vi "Temperature Feedback.vi"(10 "Temp Array":dbl[](array[numeric]), 11 "input cluster":T1) -> (3 "Change in Reactivity":dbl)   [LabVIEW 2019]
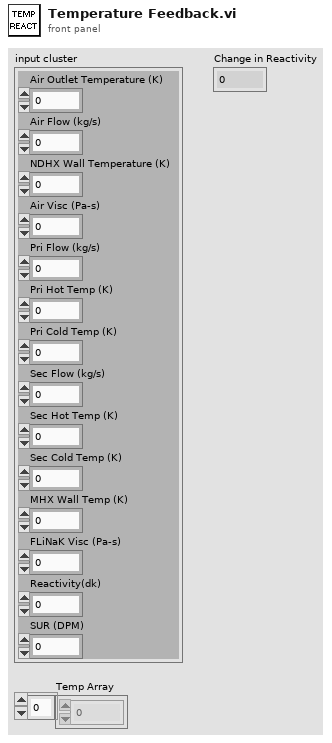
[diagram p1: front panel]
types:
  T1 = cluster{"Air Outlet Temperature (K)":dbl, "Air Flow (kg/s)":dbl, "NDHX Wall Temperature (K)":dbl, "Air Visc (Pa-s)":dbl, "Pri Flow (kg/s)":dbl, "Pri Hot Temp (K)":dbl, "Pri Cold Temp (K)":dbl, "Sec Flow (kg/s)":dbl, "Sec Hot Temp (K)":dbl, "Sec Cold Temp (K)":dbl, "MHX Wall Temp (K)":dbl, "FLiNaK Visc (Pa-s)":dbl, "Reactivity(dk)":dbl, "SUR (DPM)":dbl}
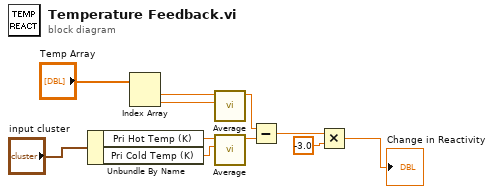
[diagram p0: block diagram]
diagram:
  n1 = Unbundle By Name("input cluster") -> ("Pri Hot Temp (K)"=w3:dbl, "Pri Cold Temp (K)"=w4:dbl)
  n2 = Index Array(array="Temp Array") -> (element #1=w10:dbl, element #2=w11:dbl)  [unwired: 2 in]
  n3 = call "Average.vi"("Number 2"=w11, "Number 1"=w10) -> ("Average"=w8:dbl)  [unwired: 9 in]
  n4 = call "Average.vi"("Number 2"=w4, "Number 1"=w3) -> ("Average"=w5:dbl)  [unwired: 9 in]
  n5 = Subtract(x=w8, y=w5) -> (x-y=w6:dbl)
  n6 = Multiply(x=w6, y=-3.0) -> (x*y=→"Change in Reactivity":dbl)
